vi "Perform Work.vi"(4 "Controller name":string, 6 "Last request":bool, 7 "Update period":dbl, 8 "error in (no error)":errorcluster, 9 "Initialize":bool, 11 "Measure Object in":refnum<class "Worker Actor.lvclass">) -> (0 "error out":errorcluster, 3 "Measure Object out":refnum<class "Worker Actor.lvclass">)   [LabVIEW 2024, in "Worker Actor.lvclass"]
uses:
  Worker Actor.lvclass
  D:/GitHub/LabActor/Template Module/Template Module.lvclass
  C:/Program Files/National Instruments/LabVIEW 2024/vi.lib/ActorFramework/Actor/Actor.lvclass
  Worker Actor.lvclass/Worker Actor.ctl
  NHMFL_Core/Libraries/Instruments/Results/Acquired Result/Acquired Result.lvclass/Acquired Result.ctl
  Template Module/Template Module.lvclass/Template Module.ctl
  Publish-Subscribe/Context.ctl
  <vilib>/ActorFramework/Actor/Actor.lvclass/Actor.ctl
  Publish-Subscribe/Interfaces/Subscriber Messages/Information Msg/Information Msg.lvclass/Information Msg.ctl
  <vilib>/ActorFramework/Message Enqueuer/Message Enqueuer.lvclass/Message Enqueuer.ctl
  Pulse Recorders/Pulse Recorder Messages/Wait for Data Msg/Wait for Result Msg.lvclass/Wait for Result Msg.ctl
  Write Done.vi
  NHMFL_Core/Libraries/Instruments/Results/Acquired Result/Read Final.vi
  Template Module/Read Name.vi
  NHMFL_Core/Libraries/Instruments/Results/Acquired Result/Write Sender.vi
  NHMFL_Core/Libraries/Instruments/Results/Acquired Result/Write Cycle count.vi
  Read Check again delay.vi
  Template Module/Read State.vi
  <vilib>/ActorFramework/Message Enqueuer/Enqueue.vi
  <vilib>/ActorFramework/Message Enqueuer/Init from Existing Queue.vi
  NHMFL_Core/Libraries/Instruments/Results/Acquired Result/Acquired Result.lvclass
  D:/GitHub/LabActor/Publish-Subscribe/Interfaces/Information/Information.lvclass
  Publish-Subscribe/Interfaces/Subscriber Messages/Information Msg/Information Msg.lvclass
  C:/Program Files/National Instruments/LabVIEW 2024/vi.lib/ActorFramework/Message/Message.lvclass
  Pulse Recorders/Pulse Recorder Messages/Wait for Data Msg/Wait for Result Msg.lvclass
  <vilib>/ActorFramework/Message Priority Queue/Priority Enqueue.vi
  <vilib>/ActorFramework/Time-Delayed Send Message/Time-Delayed Send Message.vi
  <vilib>/ActorFramework/Message Enqueuer/Message Enqueuer.lvclass
  <vilib>/ActorFramework/Actor/Actor.lvclass
  Template Module Messages/Result Reply Msg/Result Reply Msg.lvclass
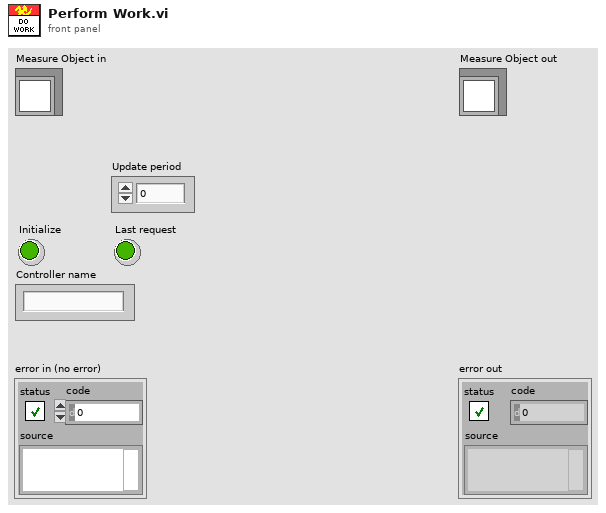
[diagram p1: front panel]
types:
  T1 = typedef "Worker State.ctl" = enum16{"Idle", "Starting", "Working", "Stopping"}
  T2 = typedef "Context.ctl" = cluster{"Topic":string, "Source":string}
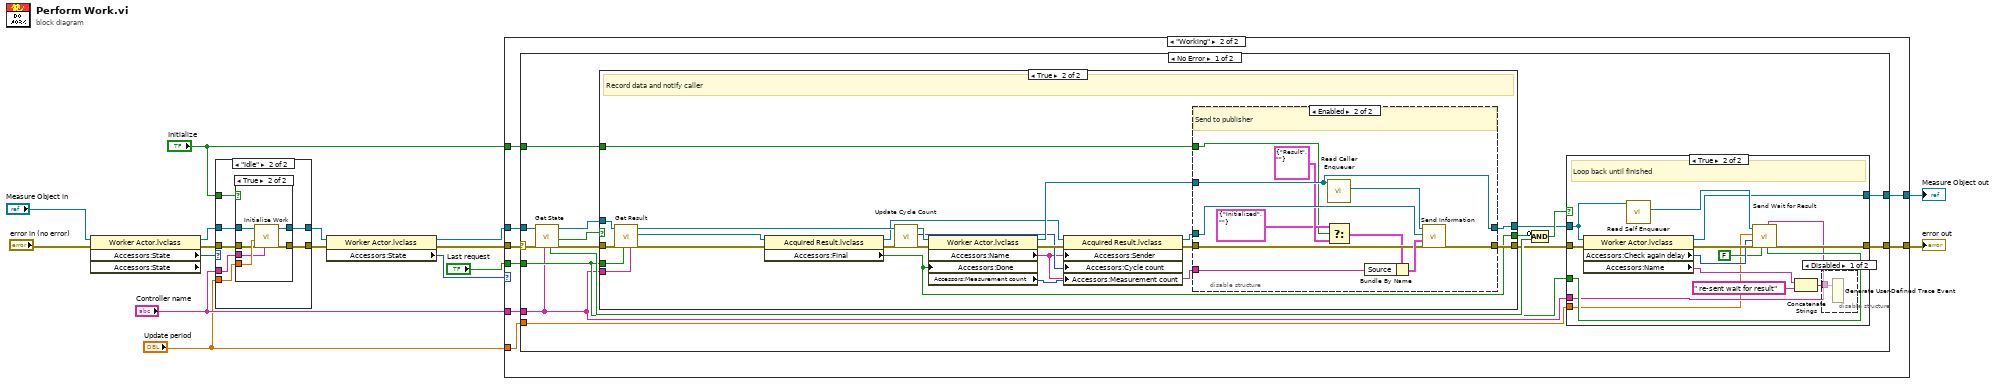
[diagram p0: block diagram]
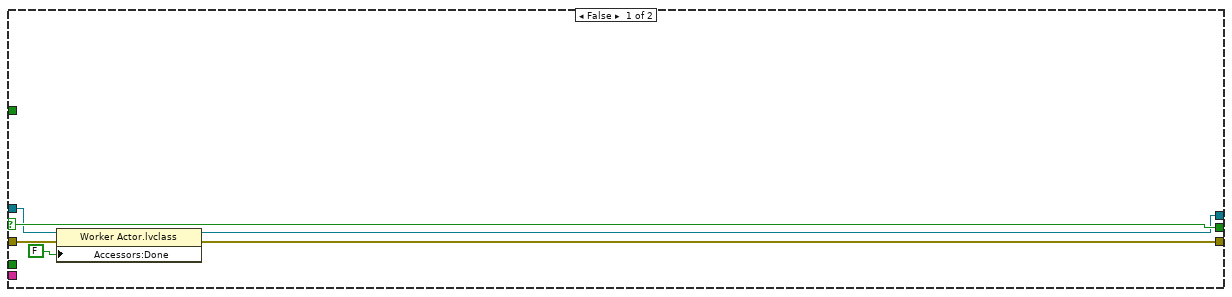
[diagram p7: hidden frame]
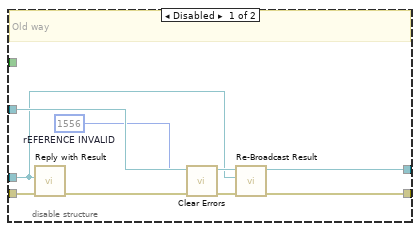
[diagram p8: hidden frame]
diagram:
  n1 = property class="Worker Actor.lvclass" props=["Accessors:State", "Accessors:State"](reference="Measure Object in", error in="error in (no error)") -> (reference out=w6:refnum<class "Worker Actor.lvclass">, error out=w2:errorcluster, "Accessors:State"=w8:T1)  [unwired: 1 out]
  n2 = case shown="\"Idle\"" w8 {
    tunnel: w2 -> [w17 w25]
    tunnel: "Initialize" -> [_ w24]
    tunnel: "Controller name" -> [_ w23]
    tunnel: "Update period" -> [_ w22]
    tunnel: w6 -> [w18 w21]
    tunnel: [w18 w20] -> w5
    tunnel: [w17 w19] -> w4
    frame "Working", Default {
    }
    frame "Idle" {
      n3 = case shown="True" w24 {
        tunnel: w21 -> [w27 w33]
        tunnel: w22 -> [_ w32]
        tunnel: w25 -> [w26 w31]
        tunnel: w23 -> [_ w30]
        tunnel: [w27 w29] -> w20
        tunnel: [w26 w28] -> w19
        frame False {
        }
        frame True {
          n4 = call-dynamic "Initialize Work.vi"("Controller name"=w30, "error in (no error)"=w31, "Update period"=w32, "Worker in"=w33) -> ("error out"=w28:errorcluster, "Worker out"=w29:refnum<class "Worker Actor.lvclass">)  [unwired: 6 in]
        }
      }
    }
  }
  n5 = property class="Worker Actor.lvclass"(reference=w5, error in=w4) -> (reference out=w9:refnum<class "Worker Actor.lvclass">, error out=w3:errorcluster, "Accessors:State"=w14:T1)
  n6 = case shown="\"Working\"" w14 {
    tunnel: w3 -> [w35 w43]
    tunnel: [w35 w42] -> w16
    tunnel: [w34 w41] -> w15
    tunnel: w9 -> [w34 w40]
    tunnel: "Last request" -> [_ w39]
    tunnel: "Initialize" -> [_ w38]
    tunnel: "Controller name" -> [_ w37]
    tunnel: "Update period" -> [_ w36]
    frame "Idle", Default {
    }
    frame "Working" {
      n7 = case shown="No Error" w43 {
        selector: w43 -> [w45 w125]
        tunnel: [w50 w125] -> w42
        tunnel: [w51 w124] -> w41
        tunnel: w40 -> [w46 w124]
        tunnel: w39 -> [w49 _]
        tunnel: w38 -> [w44 _]
        tunnel: w37 -> [w48 _]
        tunnel: w36 -> [w47 _]
        frame No Error {
          n8 = call-dynamic "Get State.vi"("Controller name"=w48, "error in (no error)"=w45, "Worker in"=w46) -> ("error out"=w58:errorcluster, "Result ready"=w59:bool, "Worker out"=w57:refnum<class "Worker Actor.lvclass">, "Check again"=w55:bool)  [unwired: 4 in, 1 out]
          n9 = case shown="True" w59 {
            selector: w59 -> [w81 _]
            tunnel: w57 -> [w79 w104]
            tunnel: w58 -> [w82 w103]
            tunnel: [w80 w97] -> w53
            tunnel: [w78 w96] -> w52
            tunnel: [w81 w87] -> w56
            tunnel: w49 -> [_ w95]
            tunnel: w48 -> [_ w86]
            tunnel: w44 -> [_ w84]
            frame False {
              n10 = property class="Worker Actor.lvclass"(reference=w79, error in=w82, "Accessors:Done"=FALSE ("Done")) -> (reference out=w78:refnum<class "Worker Actor.lvclass">, error out=w80:errorcluster)
            }
            frame True {
              # "Record data and notify caller"
              n11 = call-dynamic "Get Result.vi"("Controller name"=w86, "Last request"=w95, "error in (no error)"=w103, "Worker in"=w104) -> ("error out"=w100:errorcluster, "Result"=w89:refnum<class "Acquired Result.lvclass">, "Worker out"=w93:refnum<class "Worker Actor.lvclass">)  [unwired: 5 in]
              n12 = property class="Acquired Result.lvclass"(reference=w89, error in=w100) -> (reference out=w88:refnum<class "Acquired Result.lvclass">, error out=w90:errorcluster, "Accessors:Final"=w87:bool)
              n13 = call-dynamic "Update Cycle Count.vi"("error in (no error)"=w90, "Worker in"=w93) -> ("error out"=w94:errorcluster, "Last cycle count out"=w91:i32, "Worker out"=w92:refnum<class "Worker Actor.lvclass">)  [unwired: 7 in]
              n14 = property class="Worker Actor.lvclass"(reference=w92, error in=w94, "Accessors:Done"=w87) -> (reference out=w99:refnum<class "Worker Actor.lvclass">, error out=w102:errorcluster, "Accessors:Name"=w85:string, "Accessors:Measurement count"=w83:i32)
              n15 = property class="Acquired Result.lvclass"(reference=w88, error in=w102, "Accessors:Sender"=w85, "Accessors:Cycle count"=w91, "Accessors:Measurement count"=w83) -> (reference out=w98:refnum<class "Acquired Result.lvclass">, error out=w101:errorcluster)
              n16 = disable-structure shown="Enabled" {
                disable-tunnel: w101 -> [w112 w118]
                disable-tunnel: w99 -> [w111 w122]
                disable-tunnel: w98 -> [w110 w120]
                disable-tunnel: [w108 w117] -> w97
                disable-tunnel: [w107 w122] -> w96
                disable-tunnel: w85 -> [_ w123]
                disable-tunnel: w84 -> [_ w114]
                frame Disabled {
                  w105 = 1556  # rEFERENCE INVALID
                  # "Old way"
                  n17 = call-dynamic "Reply with Result.vi"("error in (no error)"=w112, "Result"=w110) -> ("error out"=w109:errorcluster)  [unwired: 8 in, 1 out]
                  n18 = call <vilib>:"Clear Errors.vi"("error in (no error)"=w109, "specific error code to clear (0: all)"=w105) -> ("error out"=w106:errorcluster)  [unwired: 4 in, 1 out]
                  n19 = call-dynamic "Re-Broadcast Result.vi"("error in (no error)"=w106, "Acquired Result.lvclass"=w110, "Measure Object in"=w111) -> ("error out"=w108:errorcluster, "Measure Object out"=w107:refnum<class "Worker Actor.lvclass">)  [unwired: 7 in]
                }
                frame Enabled {
                  # "Send to publisher"
                  n20 = call <vilib>:"Read Caller Enqueuer.vi"("Actor"=w122) -> ("Caller Enqueuer"=w121:refnum<class "Message Enqueuer.lvclass">)  [unwired: 10 in]
                  n21 = Select(t=T2 {"Topic"="Initialized", "Source"=""} ("Context"), s=w114, f=T2 {"Topic"="Result", "Source"=""} ("Context")) -> (s? t:f=w113:T2)
                  n22 = Bundle By Name(cluster=w113, "Source"=w123) -> (w119:T2)
                  n23 = call "Send Information.vi"("error in (no error)"=w118, "Context"=w119, "Information"=w120, "Message Enqueuer"=w121) -> ("error out"=w117:errorcluster)  [unwired: 6 in, 1 out]
                }
              }
            }
          }
          n24 = Compound Arithmetic op=AND(invert w56, w55) -> (w54:bool)
          n25 = case shown="True" w54 {
            tunnel: w52 -> [w60 w73]
            tunnel: w53 -> [w61 w70]
            tunnel: [w61 w74] -> w50
            tunnel: [w60 w68] -> w51
            tunnel: w49 -> [_ w66]
            tunnel: w48 -> [_ w64]
            tunnel: w47 -> [_ w62]
            frame False {
            }
            frame True {
              # "Loop back until finished"
              n26 = property class="Worker Actor.lvclass"(reference=w73, error in=w70) -> (reference out=w68:refnum<class "Worker Actor.lvclass">, error out=w69:errorcluster, "Accessors:Check again delay"=w65:i32, "Accessors:Name"=w67:string)
              n27 = call <vilib>:"Read Self Enqueuer.vi"("Actor"=w73) -> ("Self Enqueuer"=w75:refnum<class "Message Enqueuer.lvclass">)  [unwired: 10 in]
              n28 = call "Send Wait for Result.vi"("Last request"=w66, "Controller name"=w64, "Initialize"=FALSE, "error in (no error)"=w69, "Milliseconds To Wait"=w65, "Update period"=w62, "Message Enqueuer"=w75) -> ("error out"=w74:errorcluster)  [unwired: 2 in, 2 out]
              n29 = Concatenate Strings(w67, " re-sent wait for result" ("string")) -> (w71:string)
              n30 = disable-structure shown="Disabled" {
                disable-tunnel: w71 -> [w76 _]
                frame Disabled {
                  n31 = Generate User-Defined Trace Event(2:w76) -> ()  [unwired: 1 in]
                }
                frame Enabled {
                }
              }
            }
          }
        }
        frame Error {
        }
      }
    }
  }
  "error out" <- w16
  "Measure Object out" <- w15
